vi "Get File scan values.vi"(0 "Device":string, 5 "Variable":string, 7 "Scan/Command":string, 9 "Values: Shots#":string, 11 "error in (no error)":errorcluster) -> (4 "File scan values":dbl[](array[numeric]), 6 "values":string[](array[string]), 15 "error out":errorcluster)   [LabVIEW 2020]
doc: "This vi used to calculate array of file scan values.\nConfiguration File scan test file format is follows:\nDevice=\"SimCam\"\nVariable=\"gain\"\nValues:#shots = \"1:2,2:2,3:5\"\n\nArray of values calculated {1,1,2,2,3,3,3,3,3}"
uses:
  <vilib>/regexp/Match Regular Expression.xnode
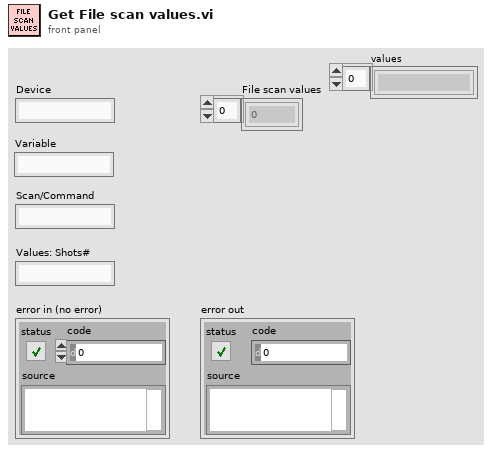
[diagram p1: front panel]
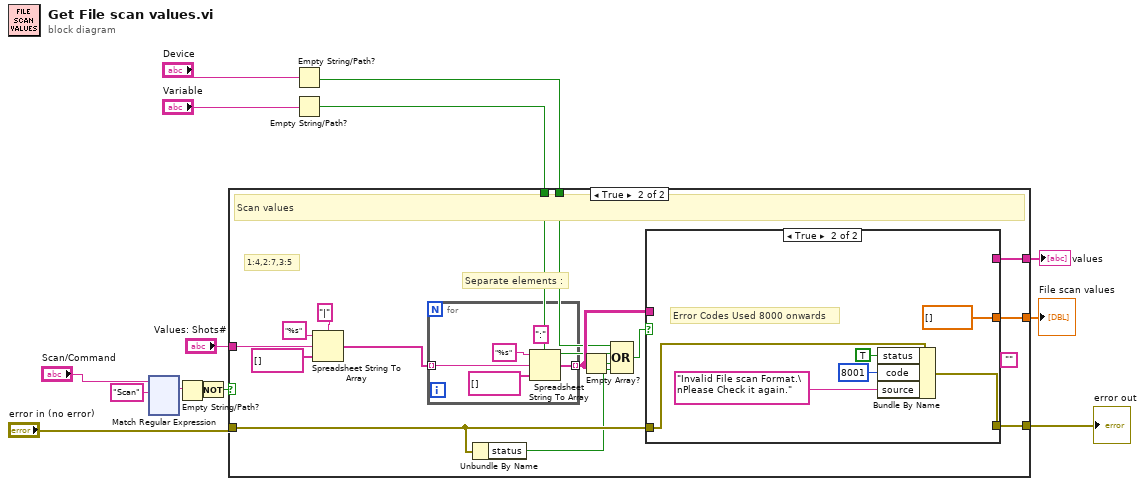
[diagram p0: block diagram]
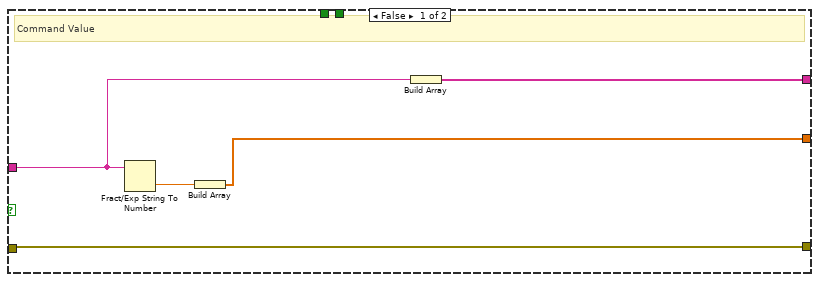
[diagram p2: hidden frame]
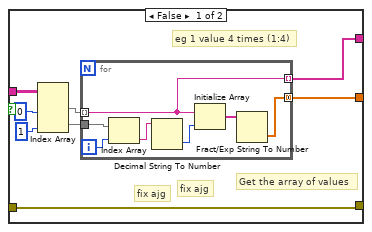
[diagram p3: hidden frame]
diagram:
  n1 = xnode "Match Regular Expression"("input string"="Scan/Command", "regular expression"="Scan") -> ("whole match"=w8:string)  [unwired: 4 in, 4 out]
  n2 = Empty String/Path?(string/path=w8) -> (empty?=w9:bool)
  n3 = Not(x=w9) -> (.not. x?=w10:bool)
  n4 = Empty String/Path?(string/path="Device") -> (empty?=w6:bool)
  n5 = Empty String/Path?(string/path="Variable") -> (empty?=w5:bool)
  n6 = case shown="True" w10 {
    tunnel: [w19 w33] -> w3
    tunnel: "error in (no error)" -> [w19 w32]
    tunnel: w5 -> [_ w28]
    tunnel: w6 -> [_ w27]
    tunnel: "Values: Shots#" -> [w16 w26]
    tunnel: [w17 w25] -> w11
    tunnel: [w15 w20] -> w1
    frame False {
      # "Command Value"
      n7 = Fract/Exp String To Number(string=w16) -> (number=w18:dbl)  [unwired: 3 in, 1 out]
      n8 = Build Array(w18) -> (w17:dbl[])
      n9 = Build Array(w16) -> (w15:string[])
    }
    frame True {
      (unwired) ""
      # "Separate elements :"
      # "1:4,2:7,3:5"
      # "Scan values"
      n10 = Spreadsheet String To Array(delimiter (Tab)="|", format string="%s", spreadsheet string=w26, array type (2D Dbl)=string[] []) -> (array=w21:string[])
      n11 = for {
        tunnel: w21 -> [w57] mode=indexing
        tunnel: [w56] -> w34 mode=indexing
        n12 = Spreadsheet String To Array(delimiter (Tab)=":", format string="%s", spreadsheet string=w57, array type (2D Dbl)=string[] []) -> (array=w56:string[])
      }
      n13 = Unbundle By Name(w32) -> ("status"=w30:bool)
      n14 = Empty Array?(array=w34) -> (empty?=w31:bool)
      n15 = Compound Arithmetic op=OR(w27, w28, w31, w30) -> (w29:bool)
      n16 = case shown="True" w29 {
        tunnel: w34 -> [w38 _]
        tunnel: w32 -> [w37 w53]
        tunnel: [w37 w51] -> w33
        tunnel: [w36 dbl[] []] -> w25
        tunnel: [w35 _] -> w20
        frame False {
          # "fix ajg"
          # "fix ajg"
          # "eg 1 value 4 times (1:4)"
          # "Get the array of values"
          n17 = Index Array(array=w38, index (col) #1=0 ("disabled index (col)"), index (col) #2=1 ("index (col)")) -> (element #1=w40:string[], element #2=w39:string[])  [unwired: 2 in]
          n18 = for {
            tunnel: w40 -> [w43] mode=indexing
            tunnel: w39 -> [w49]
            tunnel: [w44] -> w36 mode=concatenating
            tunnel: [w43] -> w35 mode=indexing
            i -> [w45]
            n19 = Index Array(array=w49, index=w45) -> (element=w46:string)
            n20 = Decimal String To Number(string=w46) -> (number=w48:i32)  [unwired: 2 in, 1 out]
            n21 = Initialize Array(w43, w48) -> (w47:string[])
            n22 = Fract/Exp String To Number(string=w47) -> (number=w44:dbl[])  [unwired: 3 in, 1 out]
          }
        }
        frame True {
          # "Error Codes Used 8000 onwards"
          n23 = Bundle By Name(cluster=w53, "status"=TRUE, "code"=8001, "source"="Invalid File scan Format.\nPlease Check it again." ("message")) -> (w51:errorcluster)
        }
      }
    }
  }
  "File scan values" <- w11
  "error out" <- w3
  "values" <- w1
